vi "Detach Bus Monitor.vi"(10 "BusMonitor":refnum<class "IBusMonitor.lvclass">, 11 "MonitoredMediator in":refnum<class "MonitoredMediator.lvclass">) -> (3 "MonitoredMediator out":refnum<class "MonitoredMediator.lvclass">)   [LabVIEW 2017, in "MonitoredMediator.lvlib" / "MonitoredMediator.lvclass"]
uses:
  MonitoredMediator.lvclass
  IBusMonitor/IBusMonitor.lvclass
  MonitoredMediator.lvclass/MonitoredMediator.ctl
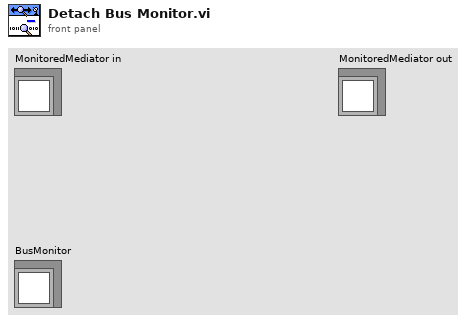
[diagram p1: front panel]
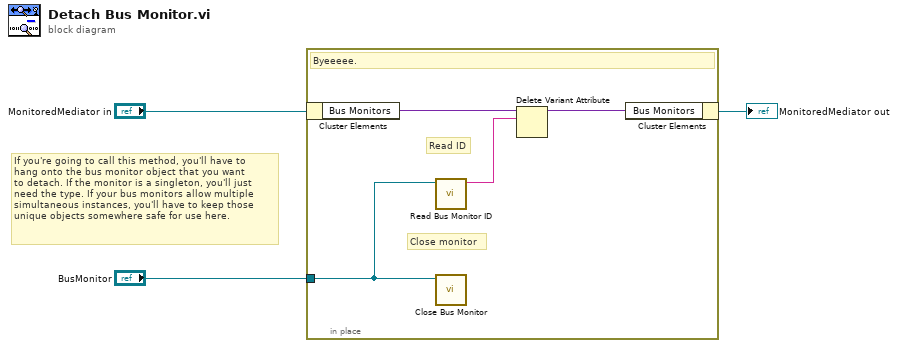
[diagram p0: block diagram]
diagram:
  # "If you're going to call this method, you'll have to\nhang onto the bus monitor object that you want\nto detach. If the monitor is a singleton, you'll just\nneed the type. If your bus monitors allow multiple\nsimultaneous instances, you'll have to keep those\nunique objects somewhere safe for use here."
  n1 = in-place {
    in-place-border: "BusMonitor" -> [w4]
    # "Read ID"
    # "Close monitor"
    # "Byeeeee."
    n2 = in-place-cluster #1("MonitoredMediator in") -> ("Bus Monitors"=w7:variant)
    n3 = call-dynamic "Read Bus Monitor ID.vi"("IBusMonitor"=w4) -> ("Bus Monitor ID"=w5:string)  [unwired: 10 in]
    n4 = call-dynamic "Close Bus Monitor.vi"("IBusMonitor In"=w4) -> ()  [unwired: 10 in, 1 out]
    n5 = Delete Variant Attribute(6:w5, 7:w7) -> (3:w6:variant)  [unwired: 1 in, 2 out]
    n6 = in-place-cluster #1("Bus Monitors"=w6) -> (→"MonitoredMediator out":refnum<class "MonitoredMediator.lvclass">)
  }
